vi "strip CRLF.vi"(4 "raw w/CRLF":string) -> (1 "CRLF stripped":string)   [LabVIEW 2011]
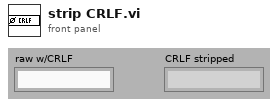
[diagram p1: front panel]
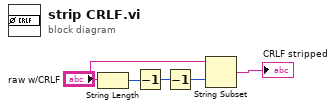
[diagram p0: block diagram]
diagram:
  n1 = String Length(string="raw w/CRLF") -> (length=w1:i32)
  n2 = Decrement(x=w1) -> (x-1=w3:i32)
  n3 = Decrement(x=w3) -> (x-1=w4:i32)
  n4 = String Subset(string="raw w/CRLF", length (rest)=w4) -> (substring=→"CRLF stripped":string)  [unwired: 1 out]
